vi "SPARK Configure Signal.vi"   [LabVIEW 2023]
doc: "Configure a signal from the SPARK."
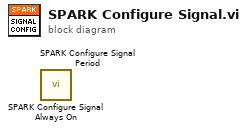
[diagram p0: block diagram]
diagram:
  n1 = call "SPARK Configure Signal Always On.vi"() -> ()  [unwired: 10 in, 2 out]
  n2 = call "SPARK Configure Signal Period.vi"() -> ()  [unwired: 10 in, 2 out]
